vi "Sold Out State_Create.vi"(0 "reference in":refnum<class "Sold Out State.lvclass">, 2 "Gum Machine.lvclass":refnum<class "Gum Machine.lvclass">, 5 "error in (no error)":errorcluster) -> (14 "reference out":refnum<class "Sold Out State.lvclass">, 19 "error out":errorcluster)   [LabVIEW 2013, in "Sold Out State.lvclass"]
doc: "Constructor."
uses:
  Sold Out State.lvclass
  Gum Machine_class/Gum Machine.lvclass
  <vilib>/addons/_AddQ/G#Object/G#Object.lvclass
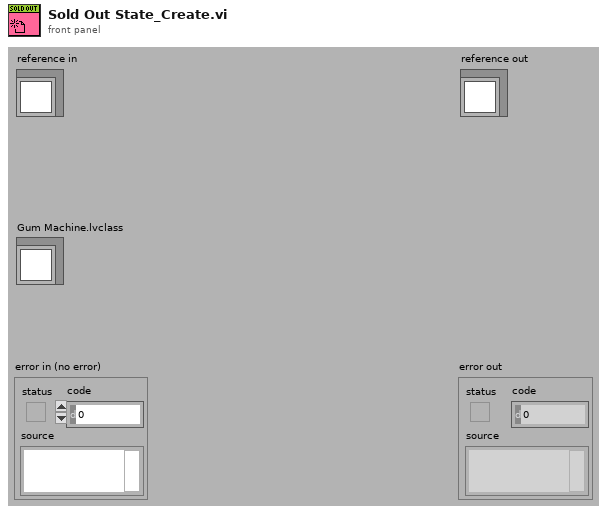
[diagram p1: front panel]
types:
  T1 = typedef "Sold Out State.lvclass/ObjectAttributesRef.ctl" = refnum<data-value>
  T2 = typedef "Sold Out State.lvclass/ObjectAttributes.ctl" = cluster{"Gum Machine.lvclass":refnum<class "Gum Machine.lvclass">}
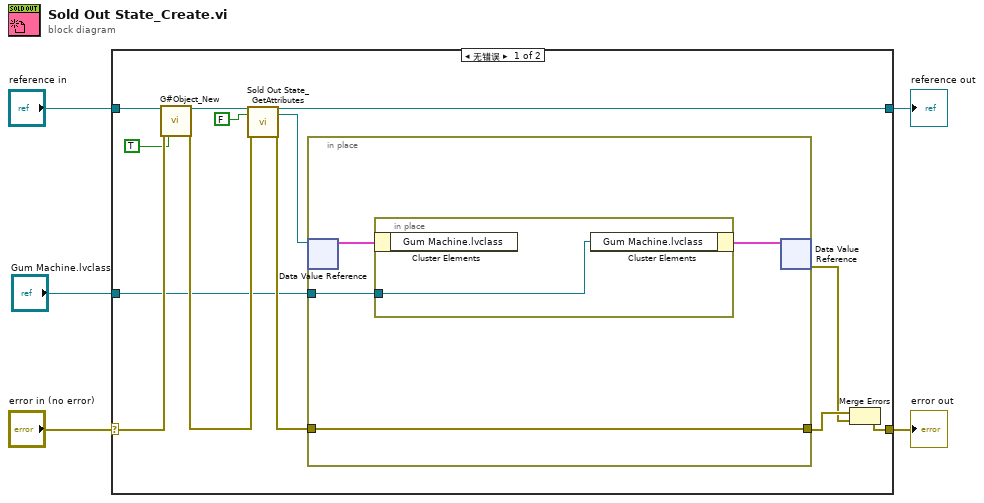
[diagram p0: block diagram]
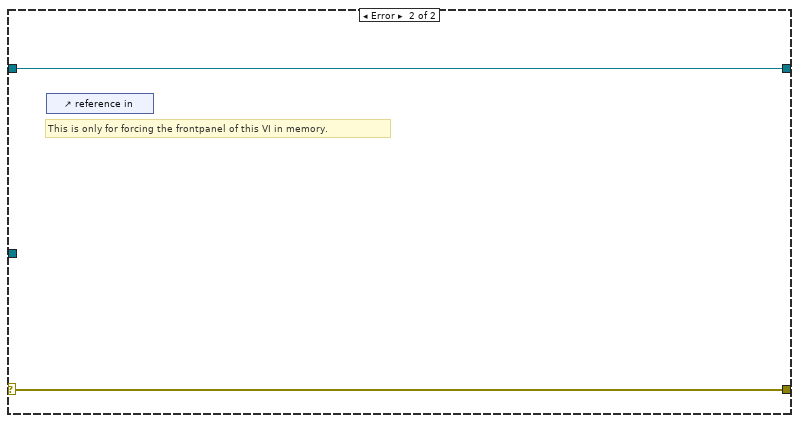
[diagram p2: hidden frame]
diagram:
  n1 = case shown="无错误" "error in (no error)" {
    selector: "error in (no error)" -> [w17 w25]
    tunnel: [w16 w25] -> w4
    tunnel: [w11 w24] -> w2
    tunnel: "reference in" -> [w18 w24]
    tunnel: "Gum Machine.lvclass" -> [w6 _]
    frame No Error {
      n2 = call <vilib>:"G#Object_New.vi"("reference in"=w18, "error in (no error)"=w17, "user counter (T)?"=TRUE ("User Counter")) -> ("reference out"=w12:refnum<class "Sold Out State.lvclass">, "error out"=w10:errorcluster)  [unwired: 14 in, 1 out]
      n3 = call "Sold Out State_GetAttributes.vi"("reference in"=w12, "return data? (T)"=FALSE ("return data"), "error in (no error)"=w10) -> ("reference out"=w11:refnum<class "Sold Out State.lvclass">, "attributes ref"=w8:T1, "error out"=w9:errorcluster)  [unwired: 13 in, 1 out]
      n4 = in-place {
        in-place-border: w9 -> [w20]
        in-place-border: [w20] -> w14
        in-place-border: w6 -> [w19]
        n5 = in-place-dvr #1(w8) -> (w21:T2)  [unwired: 1 out]
        n6 = in-place {
          in-place-border: w19 -> [w23]
          n7 = in-place-cluster #2(w21) -> ()  [unwired: 1 out]
          n8 = in-place-cluster #2("Gum Machine.lvclass"=w23) -> (w22:T2)
        }
        n9 = in-place-dvr #1(w22) -> (w13:errorcluster)  [unwired: 1 out]
      }
      n10 = Merge Errors(w14, w13) -> (w16:errorcluster)
    }
    frame Error {
      # "This is only for forcing the frontpanel of this VI in memory."
      n11 = control-ref of="reference in"() -> ()  [unwired: 1 out]
    }
  }
  "error out" <- w4
  "reference out" <- w2
